vi "SRV_VIG - Connection ID.vi"(6 "Method (Get)":enum16{"Get", "Set"}(ring), 8 "error in (no error)":errorcluster, 11 "Connection ID":refnum<k5>) -> (0 "error out":errorcluster, 3 "Connection ID out":refnum<k5>)   [LabVIEW 2009]
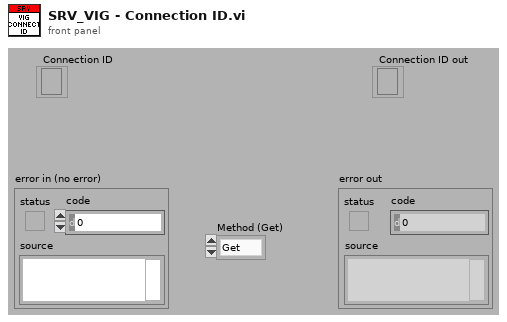
[diagram p1: front panel]
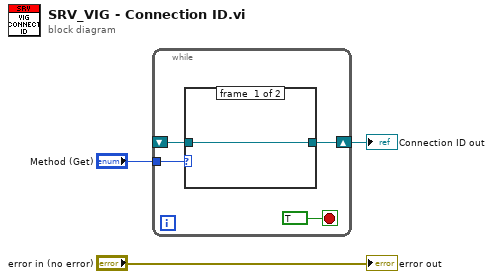
[diagram p0: block diagram]
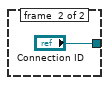
[diagram p2: hidden frame]
diagram:
  n1 = while {
    tunnel: "Method (Get)" -> [w7]
    shift-right: [w5] -> w2
    shift-left: _ -> [w6]
    stop <- TRUE stop-if-true
    n2 = case shown="\"Set\"" w7 {
      tunnel: w6 -> [w8 _]
      tunnel: [w8 "Connection ID"] -> w5
      frame #0 {
      }
      frame #1 {
      }
    }
  }
  "Connection ID out" <- w2
  "error out" <- "error in (no error)"
